vi "Get Related Window_KT.vi"(6 "Relationship":T1(ring), 9 "hWnd":u32) -> (1 "hWnd related":u32, 3 "hWnd dup":u32)   [LabVIEW 2017, in "KTools.lvlib"]
doc: "<---------Get Related Window----------->\nReturns window handle of the related window input. \ninput relation: 0=First; 1=Last; 2=Next; 3=Previous; 4=Owner; 5=Child"
uses:
  KTools.lvlib
  user32.dll
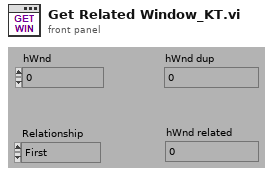
[diagram p1: front panel]
types:
  T1 = enum8{"First", "Last", "Next", "Previous", "Owner", "Child"}
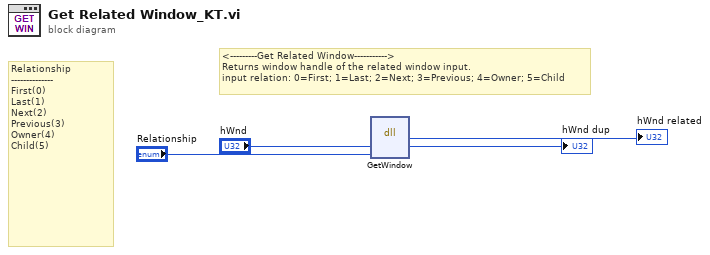
[diagram p0: block diagram]
diagram:
  # "<---------Get Related Window----------->\nReturns window handle of the related window input. \ninput relation: 0=First; 1=Last; 2=Next; 3=Previous; 4=Owner; 5=Child"
  # "Relationship\n--------------\nFirst(0)\nLast(1)\nNext(2)\nPrevious(3)\nOwner(4)\nChild(5)"
  n1 = dll-call lib="user32.dll" fn="GetWindow"("hWnd"="hWnd", "uCmd"="Relationship") -> ("hWnd related"=→"hWnd related":u32, "hWnd"=→"hWnd dup":u32)  [unwired: 4 in, 2 out]
